vi "Main Panel.vi"(10 "LVCAM":refnum<class "LVCAM.lvclass">, 11 "ABD Panel":refnum<class "ABD Panel.lvclass">) -> ()   [LabVIEW 2021, in "ABD Panel.lvclass"]
uses:
  ABD Panel.lvclass
  LVCAM/LVCAM/LVCAM/LVCAM.lvclass
  ABD Panel.lvclass/ABD Panel.ctl
  LVCAM/Msgs/LVCAM Destroy Self/LVCAM Destroy Self Msg/LVCAM Destroy Self Msg.lvclass
  C:/PPLs/LabVIEW-Composed-Actor-Model-LVCAM/LabVIEW-Composed-Actor-Model-LVCAM/LVCAM/LVCAM/Msg/Msg.lvclass
  LVCAM/LVCAM/Self Actor/Self Msg Send.vi
  LVCAM/LVCAM/Self Actor/Self Actor.lvclass
  C:/PPLs/LabVIEW-Composed-Actor-Model-LVCAM/LabVIEW-Composed-Actor-Model-LVCAM/LVCAM/Msgs/LVCAM Destroy Self/LVCAM Destroy Self Msg/LVCAM Destroy Self Msg.lvclass
  C:/PPLs/LabVIEW-Composed-Actor-Model-LVCAM/LabVIEW-Composed-Actor-Model-LVCAM/LVCAM/Msgs/LVCAM Destroy Self/LVCAM Destroy Self/LVCAM Destroy Self.lvclass
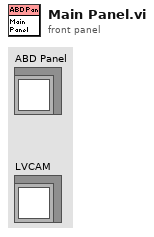
[diagram p1: front panel]
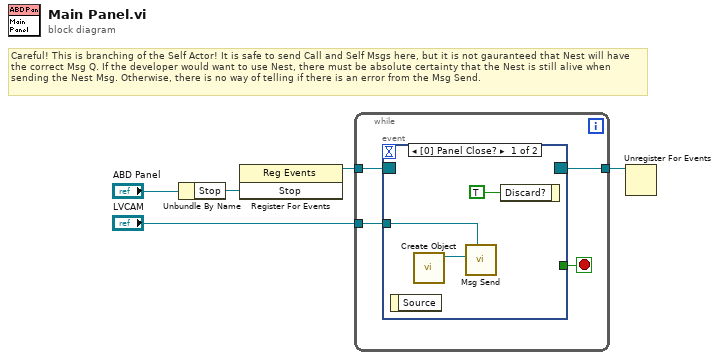
[diagram p0: block diagram]
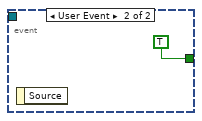
[diagram p2: hidden frame]
diagram:
  # "Careful! This is branching of the Self Actor! It is safe to send Call and Self Msgs here, but it is not gauranteed that Nest will have the correct Msg Q. If the developer would want to use Nest, there must be absolute certainty that the Nest is still alive when sending the Nest Msg. Otherwise, there is no way of telling if there is an error from the Msg Send."
  n1 = Unbundle By Name("ABD Panel") -> ("Stop"=w1:refnum<user-event>)
  n2 = register-events ("Main Register for Events")(w1) -> (reference out=w4:refnum<event-registration>)  [unwired: 2 in, 1 out]
  n3 = while {
    tunnel: w4 -> [w9]
    tunnel: [w7] -> w5
    tunnel: "LVCAM" -> [w6]
    stop <- w8 stop-if-true
    n4 = event "UI Events" shown="[0] Panel Close?" {
      selector: w9 -> [_ _]
      dyn-events: [_ _] -> w7
      timeout: _ -> [_ _]
      tunnel: [_ TRUE] -> w8
      tunnel: w6 -> [w12 _]
      event Panel Close? {
        n5 = event-data() -> ()  [unwired: 1 in, 1 out]
        n6 = call "Create Object.vi"() -> ("LVCAM Destroy Self Msg out"=w11:refnum<class "LVCAM Destroy Self Msg.lvclass">)  [unwired: 11 in]
        n7 = call-poly "Msg Send.vi"("Self Actor"=w12, "Msg"=w11) -> ()  [unwired: 9 in, 1 out]
        n8 = event-data("Discard?"=TRUE) -> ()  [unwired: 1 in, 1 out]
      }
      event User Event {
        n9 = event-data() -> ()  [unwired: 1 in, 1 out]
      }
    }
  }
  n10 = Unregister For Events(event registration refnum=w5) -> ()  [unwired: 1 in, 1 out]
